vi "Stop Core.vi"(10 "final error code":i32, 11 "CS++DeviceGUIActor in":refnum<class "CS++FgenGui.lvclass">) -> (3 "CS++DeviceGUIActor out":refnum<class "CS++FgenGui.lvclass">)   [LabVIEW 2013, in "CS++FgenGui.lvlib" / "CS++FgenGui.lvclass"]
doc: "(<B>Filename</B>: Actor Framework.lvlib:Actor.lvclass:Stop Core.vi)\n\nDefines what the actor does before it stops. Use the <B>final error code</B> input to determine whether the actor shut down in response to an error.\n\nBy default, this method does nothing. A descendant class may override it to define behavior, such as shutting down any processes the actor initiated in its override of the Actor Core method."
uses:
  CS++FgenGui.lvclass
  Core/Actors/CS++DeviceGUIActor/CS++DeviceGUIActor.lvclass
  CS++FgenGui.lvclass/CS++FgenGui.ctl
  <vilib>/ActorFramework/Message Enqueuer/Message Enqueuer.lvclass/Message Enqueuer.ctl
  <vilib>/ActorFramework/Message Enqueuer/Enqueue.vi
  <vilib>/ActorFramework/Message Priority Queue/Priority Enqueue.vi
  <vilib>/ActorFramework/Stop Msg/Stop Msg.lvclass
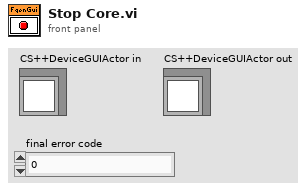
[diagram p1: front panel]
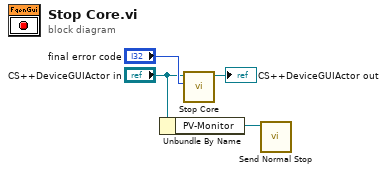
[diagram p0: block diagram]
diagram:
  n1 = Unbundle By Name("CS++DeviceGUIActor in") -> ("PV-Monitor"=w1:refnum<class "Message Enqueuer.lvclass">)
  n2 = call-parent "Stop Core.vi"("final error code"="final error code", "CS++DeviceGUIActor in"="CS++DeviceGUIActor in") -> ("CS++DeviceGUIActor out"=→"CS++DeviceGUIActor out":refnum<class "CS++FgenGui.lvclass">)  [unwired: 9 in]
  n3 = call <vilib>:"Send Normal Stop.vi"("Message Enqueuer"=w1) -> ()  [unwired: 10 in, 1 out]
